vi "linear_light_mix_tap.vi"() -> ()   [LabVIEW 2014]
panel:
  in  "maxPower (uW/mm^2)":i32
  in  "Proportion of cycles with no tap":dbl
  in  "Proportion of cycles with no light":dbl
  in  "Hold light before tap(frames)":dbl
  in  "Light on duration (frames)":dbl
  in  "Period per cycle (frames)":dbl
  in  "minPower (uW/mm^2)":i32
  in  "Taps per cycle (count)":i32
  in  "Total duration (frames)":dbl
  out "Frames":i32
  in  "Transfer and Run Date Folder After Experiment":bool
  in  "SSH user name":string
  in  "SSH password":string
  in  "Wait before recording (s)":dbl
  in  "Tags":string
  in  "Start Recording":bool
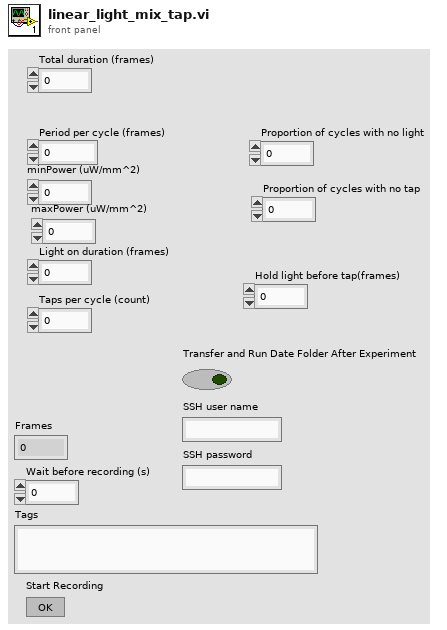
[diagram p1: front panel]
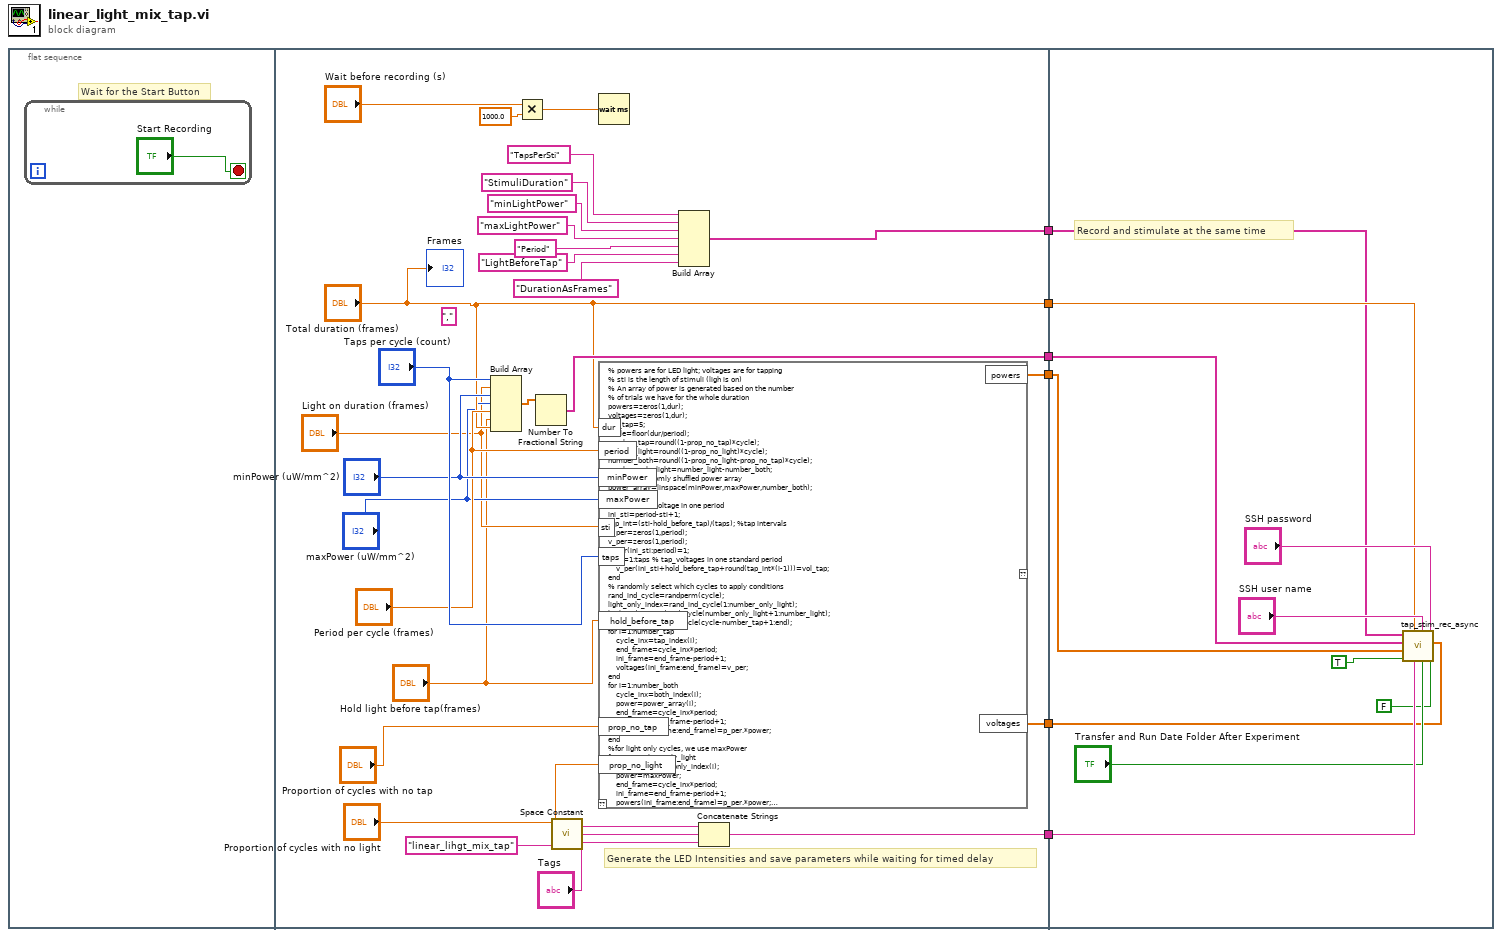
[diagram p0: block diagram]
diagram:
  n1 = flat-sequence {
    tunnel: [w32] -> w6
    tunnel: [w23] -> w5
    tunnel: ["Total duration (frames)"] -> w4
    tunnel: [w21] -> w3
    tunnel: [w17] -> w2
    tunnel: [w16] -> w1
    tunnel: w6 -> [w46]
    tunnel: w5 -> [w38]
    tunnel: w4 -> [w42]
    tunnel: w3 -> [w41]
    tunnel: w2 -> [w37]
    tunnel: w1 -> [w36]
    frame #0 {
      # "Wait for the Start Button"
      n2 = while {
        stop <- "Start Recording" stop-if-true
      }
    }
    frame #1 {
      (unwired) ","
      # "Generate the LED Intensities and save parameters while waiting for timed delay"
      n3 = Build Array("Taps per cycle (count)", "Light on duration (frames)", "minPower (uW/mm^2)", "maxPower (uW/mm^2)", "Period per cycle (frames)", "Hold light before tap(frames)", "Total duration (frames)") -> (w22:dbl[])
      n4 = Multiply(x="Wait before recording (s)", y=1000.0) -> (x*y=w30:dbl)
      n5 = Number To Fractional String(number=w22) -> (F-format string=w16:string[])  [unwired: 3 in]
      n6 = call <vilib>:"Space Constant.vi"() -> ("String"=w34:string)
      n7 = Wait (ms)(milliseconds to wait=w30) -> ()  [unwired: 1 out]
      n8 = script code="% powers are for LED light; voltages are for tapping\n% sti is the length of stimuli (ligh is on)\n% An array of power is generated based on the number\n% of trials we have for the whole duration\npowers=zeros(1,dur);\nvoltages=zeros(1,dur);\nvol_tap=5;\ncycle=floor(dur/period);\nnumber_tap=round((1-prop_no_tap)*cycle);\nnumber_light=round((1-prop_no_light)*cycle);\nnumber_both=round((1-prop_no_light-prop_no_tap)*cycle);\nnumber_only_light=number_light-number_both;\n%create randomly shuffled power array\npower_array=linspace(minPower,maxPower,number_both);\n\n% power and voltage in one period\nini_sti=period-sti+1;\ntap_int=(sti-hold_before_tap)/(taps); %tap intervals\np_per=zeros(1,period);\nv_per=zeros(1,period);\np_per(ini_sti:period)=1;\nfor i =1:taps % tap_voltages in one standard period\n    v_per(ini_sti+hold_before_tap+round(tap_int*(i-1)))=vol_tap;\nend\n% randomly select which cycles to apply conditions\nrand_ind_cycle=randperm(cycle);\nlight_only_index=rand_ind_cycle(1:number_only_light);\nboth_index=rand_ind_cycle(number_only_light+1:number_light);\ntap_index=rand_ind_cycle(cycle-number_tap+1:end);\nfor i=1:number_tap\n    cycle_inx=tap_index(i);\n    end_frame=cycle_inx*period;\n    ini_frame=end_frame-period+1;\n    voltages(ini_frame:end_frame)=v_per;\nend\nfor i=1:number_both\n    cycle_inx=both_index(i);\n    power=power_array(i);\n    end_frame=cycle_inx*period;\n    ini_frame=end_frame-period+1;\n    powers(ini_frame:end_frame)=p_per.*power;\nend\n%for light only cycles, we use maxPower\nfor i=1:number_only_light\n    cycle_inx=light_only_index(i);\n    power=maxPower;\n    end_frame=cycle_inx*period;\n    ini_frame=end_frame-period+1;\n    powers(ini_frame:end_frame)=p_per.*power;\nend"("minPower"="minPower (uW/mm^2)", "taps"="Taps per cycle (count)", "sti"="Light on duration (frames)", "period"="Period per cycle (frames)", "dur"="Total duration (frames)", "hold_before_tap"="Hold light before tap(frames)", "prop_no_tap"="Proportion of cycles with no tap", "prop_no_light"="Proportion of cycles with no light", "maxPower"="maxPower (uW/mm^2)") -> ("powers"=w21:dbl[], "voltages"=w17:dbl[])  [unwired: 1 in, 1 out]
      n9 = Build Array("TapsPerSti", "StimuliDuration", "minLightPower", "maxLightPower", "Period", "LightBeforeTap", "DurationAsFrames") -> (w23:string[])
      n10 = Concatenate Strings("linear_lihgt_mix_tap", w34, "Tags") -> (w32:string)
      "Frames" <- "Total duration (frames)"
    }
    frame #2 {
      # "Record and stimulate at the same time"
      n11 = call "tap_stim_rec_async.vi"("Convert Power to Voltage B"=FALSE, "voltages/power B"=w37, "SSH password"="SSH password", "Transfer and Run Date Folder After Experiment"="Transfer and Run Date Folder After Experiment", "SSH user name"="SSH user name", "Tags"=w46, "Frames"=w42, "Convert Power to Voltage"=TRUE, "voltages/power A"=w41, "parameters"=w36, "parameters headers"=w38) -> ()  [unwired: 1 in]
    }
  }
